vi "Write Reply Notifier.vi"(8 "error in (no error)":errorcluster, 10 "Reply Notifier":refnum<notifier>, 11 "24-Host Accepts On-Line Request from Equipment in":refnum<class "24-Host Accepts On-Line Request from Equipment.lvclass">) -> (0 "error out":errorcluster, 3 "24-Host Accepts On-Line Request from Equipment out":refnum<class "24-Host Accepts On-Line Request from Equipment.lvclass">)   [LabVIEW 2020, in "SECS Scenarios.lvlib" / "24-Host Accepts On-Line Request from Equipment.lvclass"]
uses:
  24-Host Accepts On-Line Request from Equipment.lvclass
  24-Host Accepts On-Line Request from Equipment.lvclass/24-Host Accepts On-Line Request from Equipment.ctl
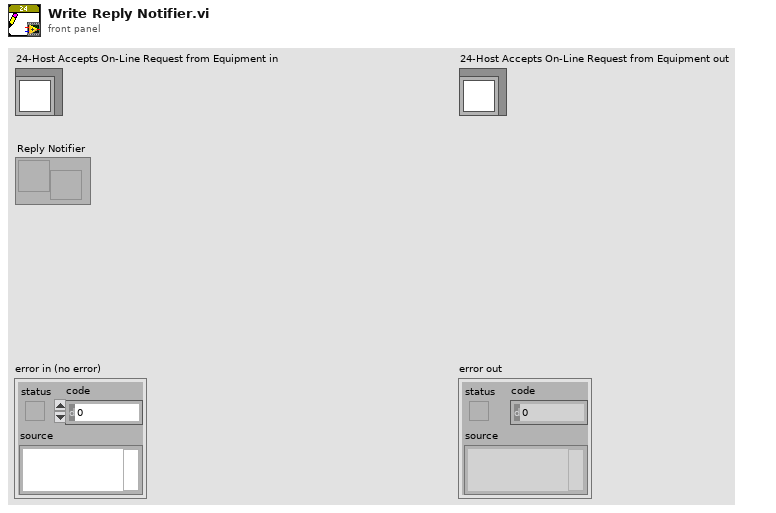
[diagram p1: front panel]
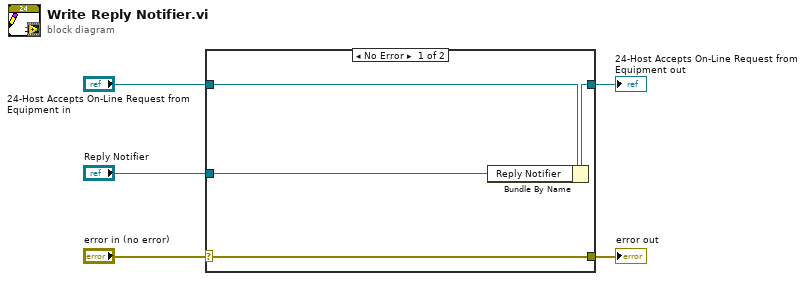
[diagram p0: block diagram]
diagram:
  n1 = case shown="No Error" "error in (no error)" {
    selector: "error in (no error)" -> [w9 w10]
    tunnel: [w9 w10] -> w4
    tunnel: [w7 w11] -> w2
    tunnel: "24-Host Accepts On-Line Request from Equipment in" -> [w8 w11]
    tunnel: "Reply Notifier" -> [w6 _]
    frame No Error {
      n2 = Bundle By Name(cluster=w8, "Reply Notifier"=w6) -> (w7:refnum<class "24-Host Accepts On-Line Request from Equipment.lvclass">)
    }
    frame Error {
    }
  }
  "error out" <- w4
  "24-Host Accepts On-Line Request from Equipment out" <- w2
